vi "Web Socket Actor Initialized.vi"(8 "error in (no error)":errorcluster, 11 "Web Socket Actor Interface in":refnum<class "Web Socket Actor Interface.lvclass">) -> (0 "error out":errorcluster, 3 "Web Socket Actor Interface out":refnum<class "Web Socket Actor Interface.lvclass">)   [LabVIEW 2020, in "Web Socket Actor Interface.lvlib" / "Web Socket Actor Interface.lvclass"]
uses:
  Web Socket Actor Interface.lvclass
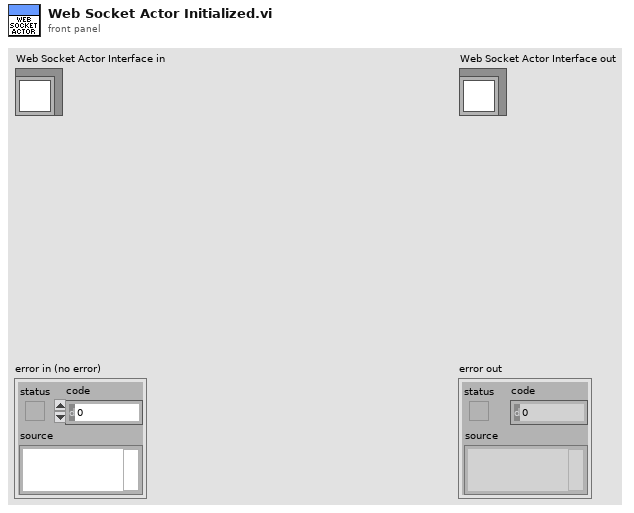
[diagram p1: front panel]
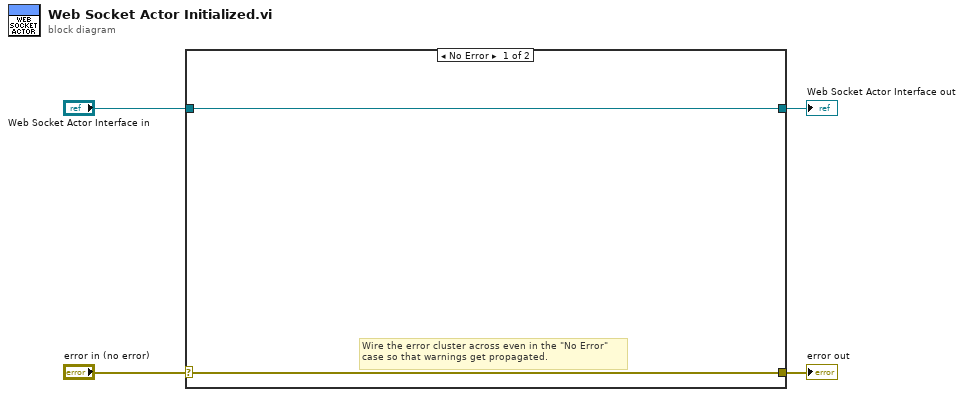
[diagram p0: block diagram]
diagram:
  n1 = case shown="No Error" "error in (no error)" {
    selector: "error in (no error)" -> [w5 w8]
    tunnel: [w5 w8] -> w3
    tunnel: [w6 w7] -> w1
    tunnel: "Web Socket Actor Interface in" -> [w6 w7]
    frame No Error {
      # "Wire the error cluster across even in the \"No Error\"\ncase so that warnings get propagated."
    }
    frame Error {
    }
  }
  "error out" <- w3
  "Web Socket Actor Interface out" <- w1
